vi "GEA2 Message Decoder.vi"(10 "GEA2 Commands and Requests":T9=enum."CMD_WRITE_SETPOINTS", 11 "Coverted Data Out":T10 {"CRC" format="%04x"; "Length" format="%02x"; "Command" format="%02x"; "Destination" format="%02x"; "Source" format="%02x"}) -> (3 "GEA Information Out":T1={"GEA Diagnostic Data - Washer"={"Speed (RPM)"=0, "Load Size"=0, "Temperature"=0, "Water Pressure"=0.0, "Detergent"=0, "Fabric Softener"=0, "Tub Direction"="", "Detergent Valve"=FALSE, "Fabric Softener Valve"=FALSE, "Recirculating Pump"=FALSE, "Drain Valve"=FALSE, "Hot Valve"=FALSE, "Cold Valve"=FALSE, "Lid Closed Status"="", "Lid Lock Status"="", "Error Count"=0, "IGBT Temperature (Deg C)"=0, "Motor Speed"=0, "Latched OOB"=0, "Raw OOB"=0, "Plaster Status"=0, "Inverter Power (W)"=0, "Target Speed(BRPM)"=0, "Latched Agitate Motor Temp (Deg C)"=0, "Current Motor Temp (Deg C)"=0, "Profiler Status"="", "Current Inverter Action"="", "Error Codes"="", "Lid Locked"=FALSE, "Lid Closed"=FALSE, "9E Diagnostic Data"={"Total Cycle Time (Min)"=0, "Total Cycle Count (Current)"=0, "Total Error Count"=0, "Machine Error History"=0, "Washer UI History"=0, "Inverter Error History"=0, "Cycle Storage Limit"=0, "Error Storage Limit"=0, "Cycle Pages Supported"=0, "Error Pages Supported"=0, "Inverter Reset Count"=0}, "9F Diagnostic Data"={"Cycle Buffer Index"="", "Page Number"="", "Total Cycle Count"=0, "Delay Start Time"=0, "Stain Selected"="", "Selected Cycle"=0, "eWash"="", "Soil Level"="", "Temperature"="", "Overnight Ready"="", "Spin Setting"="", "Control Lock Status"="", "Stain Remover"="", "Steam Assist"="", "My Cycle"="", "PreWash"="", "Debug Log Enabled"="", "Rinse"="", "Signal Level"="", "PreSoak"=""}}, "Software Version"={"Critical Major SW Version"="", "Critical Minor SW Version"="", "Major SW Version"="", "Minor SW Version"="", "Parametric Data Ver. Major"="", "Parametric Data Ver. Minor"="", "Diagnostics Data Ver. Major"="", "Diagnostics Data Ver. Minor"="", "Current Personality Setting"=""}, "Debug Search Parameters"={"Pause"=["MchStdby", "MchPz", "MchIdl", "Machine Standby", "Machine Pause", "Machine Idle"], "Run"=["MchRn", "Machine Run", "Resume Process"], "EOC"=["EOC"], "Error Codes"=["Error1", "try", "rty", "inverr"]}, "Message Count"=0, "Number of Messages"=0, "Partial Message String"="", "Full Message to Save"="", "Board ID"="", "Board Index"=0, "Source Address"=0, "Destination Address"=0, "Data to send"=[], "ReceivedData"=[], "Debug/GEA Data"=[], "Command"=0, "GEA2 Reference Out"=refnum, "GEA2 Event Registration"=refnum, "Bus Data"="", "GEA Data"=[], "Network Variable Location"=0, "Water Heater GEA2 Data"={"GEA2 Label Array"=[], "PID_PARAMETERS"=[], "SUPPORTED_MODES"=[], "Button Status"={"Switch 1"=FALSE, "Switch 2"=FALSE, "Switch 3"=FALSE, "Switch 4"=FALSE, "Switch 5"=FALSE, "Switch 6"=FALSE, "Switch 7"=FALSE, "Switch 8"=FALSE, "Switch 9"=FALSE, "Switch 10"=FALSE, "Switch 11"=FALSE, "Switch 12"=FALSE, "Switch 13"=FALSE, "Switch 14"=FALSE, "Switch 15"=FALSE, "Switch 16"=FALSE}, "Status Query"={"Days Remaining (For Std Electric and Vacation)"=0, "Unit Status"="", "Current Tank Temp in Deg F"=0, "Current Setpoint in Deg F"=0, "Filter Status (% used)"=0, "Fallback Status (Fallback heating mode)"="", "Fallback Temp"=0, "\"Set Mode\" Selection"=""}, "Service Error Codes"={"Reserved"=FALSE, "Reserved 1"=FALSE, "Reserved 2"=FALSE, "Reserved 3"=FALSE, "Reserved 4"=FALSE, "Reserved 5"=FALSE, "Reserved 6"=FALSE, "Reserved 7"=FALSE, "DataFlash Fail Status"=FALSE, "Stuck Key Fail Status"=FALSE, "Dry Tank Fail Status"=FALSE, "Miswire Fail Status"=FALSE, "Reserved 8"=FALSE, "Reserved 9"=FALSE, "Reserved 10"=FALSE, "Reserved 11"=FALSE, "UE Fail Status"=FALSE, "LE Fail Status"=FALSE, "Filter Fail Status"=FALSE, "T3A Fail Status"=FALSE, "T3B Fail Status"=FALSE, "T4 Fail Status"=FALSE, "T5 Fail Status"=FALSE, "T2 Fail Status"=FALSE, "SS Cond A Status"=FALSE, "SS Cond B Status"=FALSE, "SS Cond C Status"=FALSE, "SS Cond D Status"=FALSE, "SS Cond E Status"=FALSE, "SS Cond F Status"=FALSE, "SS Fan Status"=FALSE, "CMP Fail Status"=FALSE}, "HEM_KWH_DATA"=[], "OTHER_FAULT_COUNTS"=[], "GEA2 Raw Message"="", "Hyperterminal Data"={"Source"=0, "Destination"=0, "Command"=0, "Length"=0, "CRC"=0, "UE - state (1/0 on off)"=0, "LE - state (1/0 on off)"=0, "Comp - state (1/0 on off)"=0, "Fan  - state (1/0 on off)"=0, "Setpoint Deg F"=0, "T2(TankSensor)"=0.0, "T3A(EvapIn)"=0.0, "T3B(EvapOut)"=0.0, "T4(CompressorDischarge)"=0.0, "T5(Ambient)"=0.0, "Current"=0.0, "Voltage (Volts)"=0, "EEV Position (0-480)"=0, "Reason for last heating cycle termination"=0, "Reason Data word 1"="", "Reason Data word 2"="", "Reason Data word 3"="", "Reason Data word 4"="", "SW Debug Data"="", "Flow Events (Bit Encoded)"=0, "Heating Control Mode"=0}, "Extra Data"={"Water Capacity (Gallons)"=0, "Max Vacation Duration Days"=0, "Min Vacation Duration Days"=0, "Max Set Point (Deg F)"=0, "Min Set Point (Deg F)"=0, "T5 Resistance"=0, "T4 Resistance"=0, "T3B Resistance"=0, "T2 Resistance"=0, "STD_ELEC_RANGE"="", "SS_FAULT_COUNTS"="", "SERIAL_NUMBER"="", "READ_PERSONALITY"=0, "RQST_OVERRIDE_STATUS"="", "MODEL_SELECT_AD_VALUE"=0, "MODEL NUMBER"="", "IDLB_RESISTANCE"=0, "DSM Override Status"="", "RQST_DATA_FROM_Memory"="", "RQST_DATA_FROM_DATA_FLASH"="", "RQST_CURRENT_PID_SH_TARGET"=0, "Unit System Mode"=""}}} {"Water Heater GEA2 Data"."Hyperterminal Data"."CRC" format="%x"; "Water Heater GEA2 Data"."Hyperterminal Data"."Length" format="%x"; "Water Heater GEA2 Data"."Hyperterminal Data"."Command" format="%x"; "Water Heater GEA2 Data"."Hyperterminal Data"."Destination" format="%x"; "Water Heater GEA2 Data"."Hyperterminal Data"."Source" format="%x"; "Destination Address" format="%x"; "Source Address" format="%x"; "Command" format="%.0x"; "Data to send" format="%x"; "ReceivedData" format="%x"})   [LabVIEW 2016]
uses:
  LabVIEW GEA2 Toolkit v1.0.0.0/type defs/Data Out.ctl
  Type Definitions/GEA2 Commands.ctl
  Washer HCC/Washer HCC NEWFI/Type Definitions/ViperHawk/ViperHawk Data.ctl
  Washer HCC/Washer HCC NEWFI/Type Definitions/ViperHawk/ViperHawk Diagnostic Data.ctl
  Save File/Public/Type Definitions/Save File Software Version.ctl
  Washer HCC/Washer HCC NEWFI/Type Definitions/ViperHawk/ViperHawk Search Control.ctl
  C:/TechnologyLab/NI-2010/Trunk/Utility/LabVIEW GEA2 Toolkit v1.0.0.0/Appliance.NET/GeaCommunication.dll
  LabVIEW GEA2 Toolkit v1.0.0.0/Appliance.NET/GeaCommunication.dll
  Type Definitions/GEA2 Commands WaterHeater GEA2 Data.ctl
  Type Definitions/GEA2 Commands Button Status.ctl
  Type Definitions/GEA2 Commands Status Query.ctl
  Type Definitions/GEA2 Commands Service Error Codes.ctl
  LabVIEW GEA2 Toolkit v1.0.0.0/library/GEA2_Toolkit.lvlib
  Save File/Save File.lvlib
panel:
  in  "GEA Information In":T1={"GEA Diagnostic Data - Washer"={"Speed (RPM)"=0, "Load Size"=0, "Temperature"=0, "Water Pressure"=0.0, "Detergent"=0, "Fabric Softener"=0, "Tub Direction"="", "Detergent Valve"=FALSE, "Fabric Softener Valve"=FALSE, "Recirculating Pump"=FALSE, "Drain Valve"=FALSE, "Hot Valve"=FALSE, "Cold Valve"=FALSE, "Lid Closed Status"="", "Lid Lock Status"="", "Error Count"=0, "IGBT Temperature (Deg C)"=0, "Motor Speed"=0, "Latched OOB"=0, "Raw OOB"=0, "Plaster Status"=0, "Inverter Power (W)"=0, "Target Speed(BRPM)"=0, "Latched Agitate Motor Temp (Deg C)"=0, "Current Motor Temp (Deg C)"=0, "Profiler Status"="", "Current Inverter Action"="", "Error Codes"="", "Lid Locked"=FALSE, "Lid Closed"=FALSE, "9E Diagnostic Data"={"Total Cycle Time (Min)"=0, "Total Cycle Count (Current)"=0, "Total Error Count"=0, "Machine Error History"=0, "Washer UI History"=0, "Inverter Error History"=0, "Cycle Storage Limit"=0, "Error Storage Limit"=0, "Cycle Pages Supported"=0, "Error Pages Supported"=0, "Inverter Reset Count"=0}, "9F Diagnostic Data"={"Cycle Buffer Index"="", "Page Number"="", "Total Cycle Count"=0, "Delay Start Time"=0, "Stain Selected"="", "Selected Cycle"=0, "eWash"="", "Soil Level"="", "Temperature"="", "Overnight Ready"="", "Spin Setting"="", "Control Lock Status"="", "Stain Remover"="", "Steam Assist"="", "My Cycle"="", "PreWash"="", "Debug Log Enabled"="", "Rinse"="", "Signal Level"="", "PreSoak"=""}}, "Software Version"={"Critical Major SW Version"="", "Critical Minor SW Version"="", "Major SW Version"="", "Minor SW Version"="", "Parametric Data Ver. Major"="", "Parametric Data Ver. Minor"="", "Diagnostics Data Ver. Major"="", "Diagnostics Data Ver. Minor"="", "Current Personality Setting"=""}, "Debug Search Parameters"={"Pause"=["MchStdby", "MchPz", "MchIdl", "Machine Standby", "Machine Pause", "Machine Idle"], "Run"=["MchRn", "Machine Run", "Resume Process"], "EOC"=["EOC"], "Error Codes"=["Error1", "try", "rty", "inverr"]}, "Message Count"=0, "Number of Messages"=0, "Partial Message String"="", "Full Message to Save"="", "Board ID"="", "Board Index"=0, "Source Address"=0, "Destination Address"=0, "Data to send"=[], "ReceivedData"=[], "Debug/GEA Data"=[], "Command"=0, "GEA2 Reference Out"=refnum, "GEA2 Event Registration"=refnum, "Bus Data"="", "GEA Data"=[], "Network Variable Location"=0, "Water Heater GEA2 Data"={"GEA2 Label Array"=[], "PID_PARAMETERS"=[], "SUPPORTED_MODES"=[], "Button Status"={"Switch 1"=FALSE, "Switch 2"=FALSE, "Switch 3"=FALSE, "Switch 4"=FALSE, "Switch 5"=FALSE, "Switch 6"=FALSE, "Switch 7"=FALSE, "Switch 8"=FALSE, "Switch 9"=FALSE, "Switch 10"=FALSE, "Switch 11"=FALSE, "Switch 12"=FALSE, "Switch 13"=FALSE, "Switch 14"=FALSE, "Switch 15"=FALSE, "Switch 16"=FALSE}, "Status Query"={"Days Remaining (For Std Electric and Vacation)"=0, "Unit Status"="", "Current Tank Temp in Deg F"=0, "Current Setpoint in Deg F"=0, "Filter Status (% used)"=0, "Fallback Status (Fallback heating mode)"="", "Fallback Temp"=0, "\"Set Mode\" Selection"=""}, "Service Error Codes"={"Reserved"=FALSE, "Reserved 1"=FALSE, "Reserved 2"=FALSE, "Reserved 3"=FALSE, "Reserved 4"=FALSE, "Reserved 5"=FALSE, "Reserved 6"=FALSE, "Reserved 7"=FALSE, "DataFlash Fail Status"=FALSE, "Stuck Key Fail Status"=FALSE, "Dry Tank Fail Status"=FALSE, "Miswire Fail Status"=FALSE, "Reserved 8"=FALSE, "Reserved 9"=FALSE, "Reserved 10"=FALSE, "Reserved 11"=FALSE, "UE Fail Status"=FALSE, "LE Fail Status"=FALSE, "Filter Fail Status"=FALSE, "T3A Fail Status"=FALSE, "T3B Fail Status"=FALSE, "T4 Fail Status"=FALSE, "T5 Fail Status"=FALSE, "T2 Fail Status"=FALSE, "SS Cond A Status"=FALSE, "SS Cond B Status"=FALSE, "SS Cond C Status"=FALSE, "SS Cond D Status"=FALSE, "SS Cond E Status"=FALSE, "SS Cond F Status"=FALSE, "SS Fan Status"=FALSE, "CMP Fail Status"=FALSE}, "HEM_KWH_DATA"=[], "OTHER_FAULT_COUNTS"=[], "GEA2 Raw Message"="", "Hyperterminal Data"={"Source"=0, "Destination"=0, "Command"=0, "Length"=0, "CRC"=0, "UE - state (1/0 on off)"=0, "LE - state (1/0 on off)"=0, "Comp - state (1/0 on off)"=0, "Fan  - state (1/0 on off)"=0, "Setpoint Deg F"=0, "T2(TankSensor)"=0.0, "T3A(EvapIn)"=0.0, "T3B(EvapOut)"=0.0, "T4(CompressorDischarge)"=0.0, "T5(Ambient)"=0.0, "Current"=0.0, "Voltage (Volts)"=0, "EEV Position (0-480)"=0, "Reason for last heating cycle termination"=0, "Reason Data word 1"="", "Reason Data word 2"="", "Reason Data word 3"="", "Reason Data word 4"="", "SW Debug Data"="", "Flow Events (Bit Encoded)"=0, "Heating Control Mode"=0}, "Extra Data"={"Water Capacity (Gallons)"=0, "Max Vacation Duration Days"=0, "Min Vacation Duration Days"=0, "Max Set Point (Deg F)"=0, "Min Set Point (Deg F)"=0, "T5 Resistance"=0, "T4 Resistance"=0, "T3B Resistance"=0, "T2 Resistance"=0, "STD_ELEC_RANGE"="", "SS_FAULT_COUNTS"="", "SERIAL_NUMBER"="", "READ_PERSONALITY"=0, "RQST_OVERRIDE_STATUS"="", "MODEL_SELECT_AD_VALUE"=0, "MODEL NUMBER"="", "IDLB_RESISTANCE"=0, "DSM Override Status"="", "RQST_DATA_FROM_Memory"="", "RQST_DATA_FROM_DATA_FLASH"="", "RQST_CURRENT_PID_SH_TARGET"=0, "Unit System Mode"=""}}} {"Water Heater GEA2 Data"."Hyperterminal Data"."CRC" format="%x"; "Water Heater GEA2 Data"."Hyperterminal Data"."Length" format="%x"; "Water Heater GEA2 Data"."Hyperterminal Data"."Command" format="%x"; "Water Heater GEA2 Data"."Hyperterminal Data"."Destination" format="%x"; "Water Heater GEA2 Data"."Hyperterminal Data"."Source" format="%x"; "Destination Address" format="%x"; "Source Address" format="%x"; "Command" format="%.0x"; "Data to send" format="%x"; "ReceivedData" format="%x"}
  out "Hex Array Out":string[](array[string])
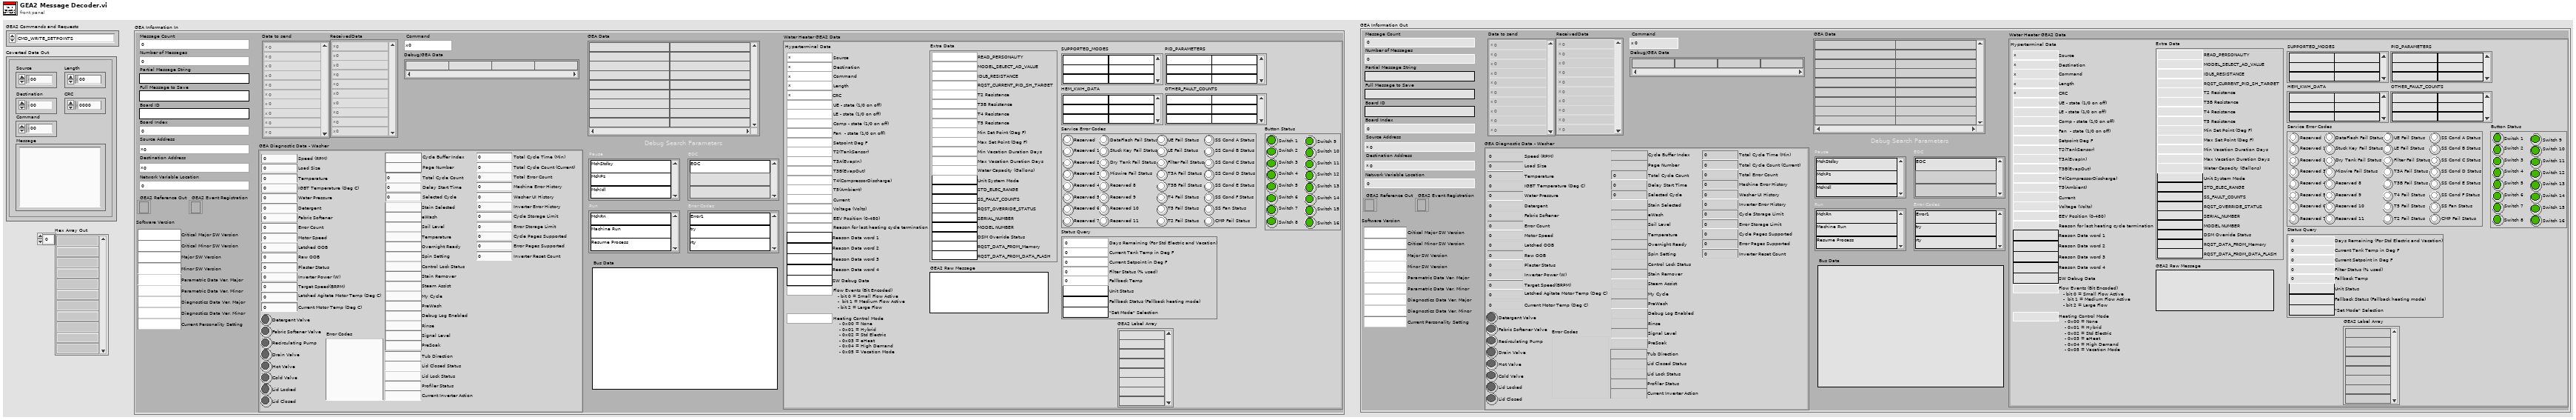
[diagram p1: front panel]
types:
  T1 = typedef "ViperHawk Data.ctl" = cluster{"GEA Diagnostic Data - Washer":T2, "Software Version":T3, "Debug Search Parameters":T4, "Message Count":i32, "Number of Messages":i32, "Partial Message String":string, "Full Message to Save":string, "Board ID":string, "Board Index":i32, "Source Address":u8, "Destination Address":u8, "Data to send":u8[], "ReceivedData":u8[], "Debug/GEA Data":string[], "Command":u8, "GEA2 Reference Out":refnum<k24>, "GEA2 Event Registration":refnum<event-registration>, "Bus Data":string, "GEA Data":string[][], "Network Variable Location":i32, "Water Heater GEA2 Data":T5}
  T2 = typedef "ViperHawk Diagnostic Data.ctl" = cluster{"Speed (RPM)":u32, "Load Size":u32, "Temperature":u32, "Water Pressure":dbl, "Detergent":u32, "Fabric Softener":u32, "Tub Direction":string, "Detergent Valve":bool, "Fabric Softener Valve":bool, "Recirculating Pump":bool, "Drain Valve":bool, "Hot Valve":bool, "Cold Valve":bool, "Lid Closed Status":string, "Lid Lock Status":string, "Error Count":u32, "IGBT Temperature (Deg C)":u32, "Motor Speed":u32, "Latched OOB":u32, "Raw OOB":u32, "Plaster Status":u32, "Inverter Power (W)":u32, "Target Speed(BRPM)":u32, "Latched Agitate Motor Temp (Deg C)":u32, "Current Motor Temp (Deg C)":u32, "Profiler Status":string, "Current Inverter Action":string, "Error Codes":string, "Lid Locked":bool, "Lid Closed":bool, "9E Diagnostic Data":cluster{"Total Cycle Time (Min)":u32, "Total Cycle Count (Current)":u16, "Total Error Count":u16, "Machine Error History":u32, "Washer UI History":u32, "Inverter Error History":u32, "Cycle Storage Limit":u8, "Error Storage Limit":u8, "Cycle Pages Supported":u8, "Error Pages Supported":u8, "Inverter Reset Count":u16}, "9F Diagnostic Data":cluster{"Cycle Buffer Index":string, "Page Number":string, "Total Cycle Count":u32, "Delay Start Time":u32, "Stain Selected":string, "Selected Cycle":u32, "eWash":string, "Soil Level":string, "Temperature":string, "Overnight Ready":string, "Spin Setting":string, "Control Lock Status":string, "Stain Remover":string, "Steam Assist":string, "My Cycle":string, "PreWash":string, "Debug Log Enabled":string, "Rinse":string, "Signal Level":string, "PreSoak":string}}
  T3 = typedef "Save File.lvlib/Save File Software Version.ctl" = cluster{"Critical Major SW Version":string, "Critical Minor SW Version":string, "Major SW Version":string, "Minor SW Version":string, "Parametric Data Ver. Major":string, "Parametric Data Ver. Minor":string, "Diagnostics Data Ver. Major":string, "Diagnostics Data Ver. Minor":string, "Current Personality Setting":string}
  T4 = typedef "ViperHawk Search Control.ctl" = cluster{"Pause":string[], "Run":string[], "EOC":string[], "Error Codes":string[]}
  T5 = typedef "GEA2 Commands WaterHeater GEA2 Data.ctl" = cluster{"GEA2 Label Array":string[], "PID_PARAMETERS":string[][], "SUPPORTED_MODES":string[][], "Button Status":T6, "Status Query":T7, "Service Error Codes":T8, "HEM_KWH_DATA":string[][], "OTHER_FAULT_COUNTS":string[][], "GEA2 Raw Message":string, "Hyperterminal Data":cluster{"Source":u8, "Destination":u8, "Command":u8, "Length":u8, "CRC":u16, "UE - state (1/0 on off)":u8, "LE - state (1/0 on off)":u8, "Comp - state (1/0 on off)":u8, "Fan  - state (1/0 on off)":u8, "Setpoint Deg F":i32, "T2(TankSensor)":dbl, "T3A(EvapIn)":dbl, "T3B(EvapOut)":dbl, "T4(CompressorDischarge)":dbl, "T5(Ambient)":dbl, "Current":dbl, "Voltage (Volts)":u16, "EEV Position (0-480)":u16, "Reason for last heating cycle termination":u16, "Reason Data word 1":string, "Reason Data word 2":string, "Reason Data word 3":string, "Reason Data word 4":string, "SW Debug Data":string, "Flow Events (Bit Encoded)":u16, "Heating Control Mode":u16}, "Extra Data":cluster{"Water Capacity (Gallons)":u32, "Max Vacation Duration Days":u32, "Min Vacation Duration Days":u32, "Max Set Point (Deg F)":u32, "Min Set Point (Deg F)":u32, "T5 Resistance":u32, "T4 Resistance":u32, "T3B Resistance":u32, "T2 Resistance":u32, "STD_ELEC_RANGE":string, "SS_FAULT_COUNTS":string, "SERIAL_NUMBER":string, "READ_PERSONALITY":u8, "RQST_OVERRIDE_STATUS":string, "MODEL_SELECT_AD_VALUE":u32, "MODEL NUMBER":string, "IDLB_RESISTANCE":u32, "DSM Override Status":string, "RQST_DATA_FROM_Memory":string, "RQST_DATA_FROM_DATA_FLASH":string, "RQST_CURRENT_PID_SH_TARGET":u16, "Unit System Mode":string}}
  T6 = typedef "GEA2 Commands Button Status.ctl" = cluster{"Switch 1":bool, "Switch 2":bool, "Switch 3":bool, "Switch 4":bool, "Switch 5":bool, "Switch 6":bool, "Switch 7":bool, "Switch 8":bool, "Switch 9":bool, "Switch 10":bool, "Switch 11":bool, "Switch 12":bool, "Switch 13":bool, "Switch 14":bool, "Switch 15":bool, "Switch 16":bool}
  T7 = typedef "GEA2 Commands Status Query.ctl" = cluster{"Days Remaining (For Std Electric and Vacation)":u8, "Unit Status":string, "Current Tank Temp in Deg F":u8, "Current Setpoint in Deg F":u8, "Filter Status (% used)":u8, "Fallback Status (Fallback heating mode)":string, "Fallback Temp":u8, "\"Set Mode\" Selection":string}
  T8 = typedef "GEA2 Commands Service Error Codes.ctl" = cluster{"Reserved":bool, "Reserved 1":bool, "Reserved 2":bool, "Reserved 3":bool, "Reserved 4":bool, "Reserved 5":bool, "Reserved 6":bool, "Reserved 7":bool, "DataFlash Fail Status":bool, "Stuck Key Fail Status":bool, "Dry Tank Fail Status":bool, "Miswire Fail Status":bool, "Reserved 8":bool, "Reserved 9":bool, "Reserved 10":bool, "Reserved 11":bool, "UE Fail Status":bool, "LE Fail Status":bool, "Filter Fail Status":bool, "T3A Fail Status":bool, "T3B Fail Status":bool, "T4 Fail Status":bool, "T5 Fail Status":bool, "T2 Fail Status":bool, "SS Cond A Status":bool, "SS Cond B Status":bool, "SS Cond C Status":bool, "SS Cond D Status":bool, "SS Cond E Status":bool, "SS Cond F Status":bool, "SS Fan Status":bool, "CMP Fail Status":bool}
  T9 = typedef "GEA2 Commands.ctl" = enum16{"CMD_CANCEL_EEV_POSITION", "CMD_CLEAR_ENERGY_USAGE_CTRS", "CMD_CLEAR_FAULT_COUNTS", "CMD_CLEAR_OVERRIDE_STATUS", "CMD_COMP_OFF", "CMD_COMP_ON", "CMD_DSM_OVERRIDES", "CMD_EEV_POSITION", "CMD_ENTER_EXIT_FCT_MODE", "CMD_ENTER_FACT_MODE", "CMD_HP_RUN_6MIN", "CMD_INITIATE_REMOTE_DSM_OVERRIDE", "CMD_LE_2_SECONDS", "CMD_REFRESH_SERVICE_TIMEOUTS", "CMD_RESET", "CMD_RESET_FILTER_TIMES", "CMD_RESTORE_EEPROM_DEFAULTS", "CMD_RQST_LED_STATUS", "CMD_SET_AMBIENT_THRESH_1", "CMD_SET_AMBIENT_THRESH_2", "CMD_SET_AMBIENT_THRESH_3", "CMD_SET_CURRENTS", "CMD_SET_EEV_DRIVE_LINES", "CMD_SET_EEV_STOP_POSITION", "CMD_SET_LEDS", "CMD_SET_MODEL_NUMBER", "CMD_SET_PID_I_DENOM_OVER_THR", "CMD_SET_PID_I_DENOM_UNDER_THR", "CMD_SET_PID_LOW_SH_TARGET", "CMD_SET_PID_MID_SH_TARGET", "CMD_SET_PID_P_DENOMINATOR", "CMD_SET_SERIAL_NUMBER", "CMD_SET_START_POS_OVER_THR", "CMD_SET_START_POS_UNDER_THR", "CMD_TOGGLE_FAN", "CMD_TOGGLE_LE_SERV", "CMD_TOGGLE_SERVICE_MODE", "CMD_TOGGLE_UE_SERV", "CMD_TURN_ON_OFF_DLB", "CMD_UE_2_SECONDS", "CMD_UPDATE_DSM_LEVEL", "CMD_UPDATE_MODE", "CMD_WRITE_SETPOINTS", "REQ_READ_KEY_STATUS", "REQ_SYSTEM_MODE", "RQST_CURRENT_PID_SH_TARGET", "RQST_DATA_FROM_DATA_FLASH", "RQST_DATA_FROM_MEMORY", "RQST_DSM_OVERRIDE_STATUS", "RQST_HEM_KWH_DATA", "RQST_HYPERTERM_OUTPUT_DATA", "RQST_IDLB_RESISTANCE", "RQST_MODEL_NUMBER", "RQST_MODEL_SELECT_AD_VALUE", "RQST_OTHER_FAULT_COUNTS", "RQST_OVERRIDE_STATUS", "RQST_PID_PARAMETERS", "RQST_READ_PERSONALITY", "RQST_SERIAL_NUMBER", "RQST_SERVICE_ERROR_CODES", "RQST_Software_Version", "RQST_SS_FAULT_COUNTS", "RQST_STATUS_QUERY", "RQST_STD_ELEC_RANGE", "RQST_SUPPORTED_MODES", "RQST_T2_RESISTANCE", "RQST_T3B_RESISTANCE", "RQST_T4_RESISTANCE", "RQST_T5_RESISTANCE", "RQST_TEMP_RANGE", "RQST_VACATION_RANGE", "RQST_WATER_CAPACITY"}
  T10 = typedef "GEA2_Toolkit.lvlib/Data Out.ctl" = cluster{"Source":u8, "Destination":u8, "Command":u8, "Length":u8, "CRC":u16, "Message":string}
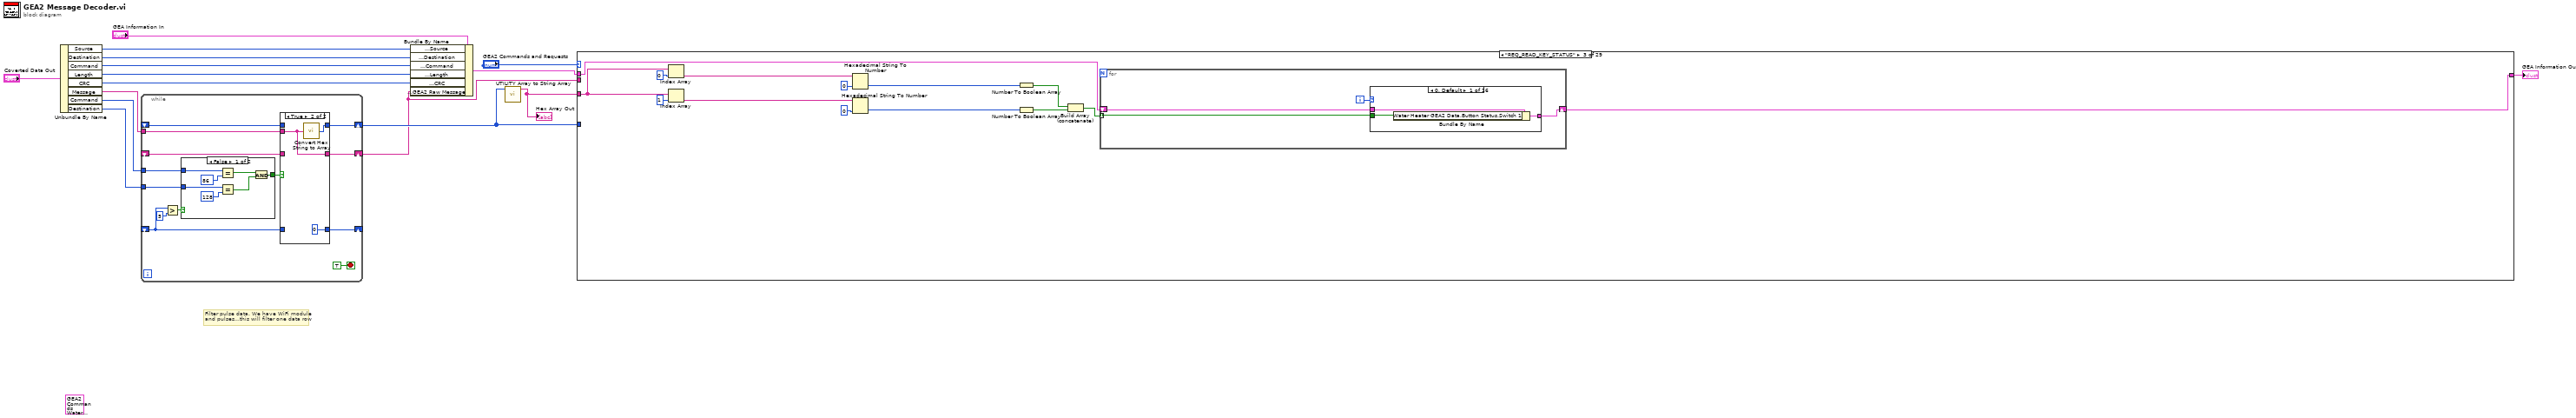
[diagram p0: block diagram]
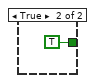
[diagram p2: hidden frame]
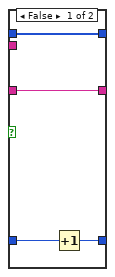
[diagram p3: hidden frame]
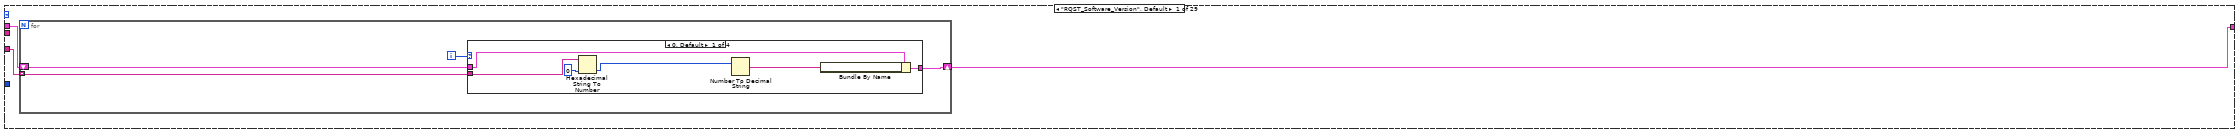
[diagram p4: hidden frame]
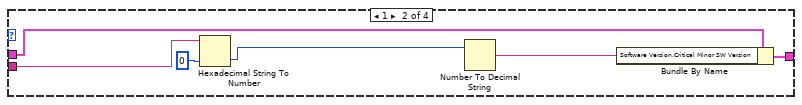
[diagram p5: hidden frame]
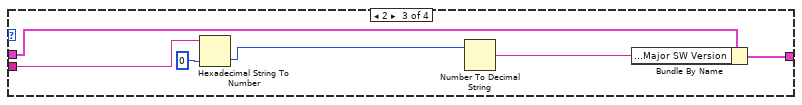
[diagram p6: hidden frame]
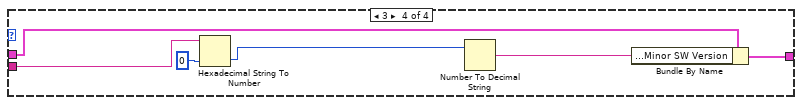
[diagram p7: hidden frame]
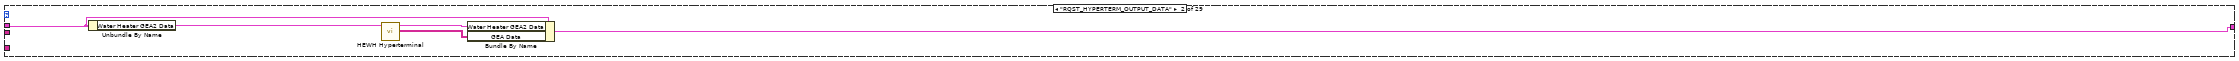
[diagram p8: hidden frame]
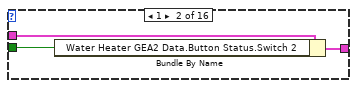
[diagram p9: hidden frame]
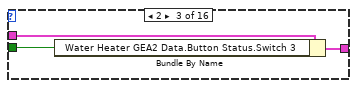
[diagram p10: hidden frame]
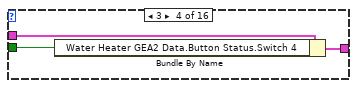
[diagram p11: hidden frame]
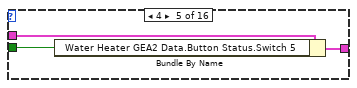
[diagram p12: hidden frame]
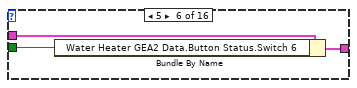
[diagram p13: hidden frame]
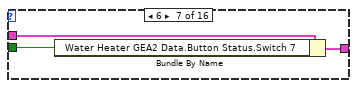
[diagram p14: hidden frame]
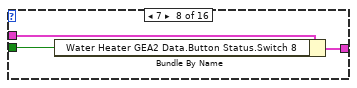
[diagram p15: hidden frame]
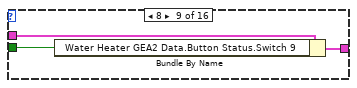
[diagram p16: hidden frame]
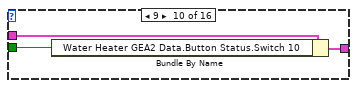
[diagram p17: hidden frame]
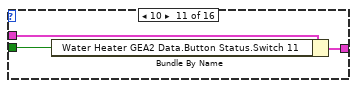
[diagram p18: hidden frame]
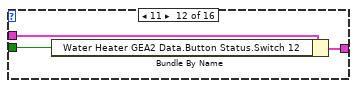
[diagram p19: hidden frame]
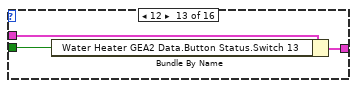
[diagram p20: hidden frame]
diagram:
  (unwired) T5 {"GEA2 Label Array"=[], "PID_PARAMETERS"=[], "SUPPORTED_MODES"=[], "Button Status"={"Switch 1"=FALSE, "Switch 2"=FALSE, "Switch 3"=FALSE, "Switch 4"=FALSE, "Switch 5"=FALSE, "Switch 6"=FALSE, "Switch 7"=FALSE, "Switch 8"=FALSE, "Switch 9"=FALSE, "Switch 10"=FALSE, "Switch 11"=FALSE, "Switch 12"=FALSE, "Switch 13"=FALSE, "Switch 14"=FALSE, "Switch 15"=FALSE, "Switch 16"=FALSE}, "Status Query"={"Days Remaining (For Std Electric and Vacation)"=0, "Unit Status"="", "Current Tank Temp in Deg F"=0, "Current Setpoint in Deg F"=0, "Filter Status (% used)"=0, "Fallback Status (Fallback heating mode)"="", "Fallback Temp"=0, "\"Set Mode\" Selection"=""}, "Service Error Codes"={"Reserved"=FALSE, "Reserved 1"=FALSE, "Reserved 2"=FALSE, "Reserved 3"=FALSE, "Reserved 4"=FALSE, "Reserved 5"=FALSE, "Reserved 6"=FALSE, "Reserved 7"=FALSE, "DataFlash Fail Status"=FALSE, "Stuck Key Fail Status"=FALSE, "Dry Tank Fail Status"=FALSE, "Miswire Fail Status"=FALSE, "Reserved 8"=FALSE, "Reserved 9"=FALSE, "Reserved 10"=FALSE, "Reserved 11"=FALSE, "UE Fail Status"=FALSE, "LE Fail Status"=FALSE, "Filter Fail Status"=FALSE, "T3A Fail Status"=FALSE, "T3B Fail Status"=FALSE, "T4 Fail Status"=FALSE, "T5 Fail Status"=FALSE, "T2 Fail Status"=FALSE, "SS Cond A Status"=FALSE, "SS Cond B Status"=FALSE, "SS Cond C Status"=FALSE, "SS Cond D Status"=FALSE, "SS Cond E Status"=FALSE, "SS Cond F Status"=FALSE, "SS Fan Status"=FALSE, "CMP Fail Status"=FALSE}, "HEM_KWH_DATA"=[], "OTHER_FAULT_COUNTS"=[], "GEA2 Raw Message"="", "Hyperterminal Data"={"Source"=0, "Destination"=0, "Command"=0, "Length"=0, "CRC"=0, "UE - state (1/0 on off)"=0, "LE - state (1/0 on off)"=0, "Comp - state (1/0 on off)"=0, "Fan  - state (1/0 on off)"=0, "Setpoint Deg F"=0, "T2(TankSensor)"=0.0, "T3A(EvapIn)"=0.0, "T3B(EvapOut)"=0.0, "T4(CompressorDischarge)"=0.0, "T5(Ambient)"=0.0, "Current"=0.0, "Voltage (Volts)"=0, "EEV Position (0-480)"=0, "Reason for last heating cycle termination"=0, "Reason Data word 1"="", "Reason Data word 2"="", "Reason Data word 3"="", "Reason Data word 4"="", "SW Debug Data"="", "Flow Events (Bit Encoded)"=0, "Heating Control Mode"=0}, "Extra Data"={"Water Capacity (Gallons)"=0, "Max Vacation Duration Days"=0, "Min Vacation Duration Days"=0, "Max Set Point (Deg F)"=0, "Min Set Point (Deg F)"=0, "T5 Resistance"=0, "T4 Resistance"=0, "T3B Resistance"=0, "T2 Resistance"=0, "STD_ELEC_RANGE"="", "SS_FAULT_COUNTS"="", "SERIAL_NUMBER"="", "READ_PERSONALITY"=0, "RQST_OVERRIDE_STATUS"="", "MODEL_SELECT_AD_VALUE"=0, "MODEL NUMBER"="", "IDLB_RESISTANCE"=0, "DSM Override Status"="", "RQST_DATA_FROM_Memory"="", "RQST_DATA_FROM_DATA_FLASH"="", "RQST_CURRENT_PID_SH_TARGET"=0, "Unit System Mode"=""}}
  # "Filter pulse data. We have WiFi module\nand pulses...this will filter one data row"
  n1 = Unbundle By Name("Coverted Data Out") -> ("Source"=w10:u8, "Destination"=w9:u8, "Command"=w8:u8, "Length"=w7:u8, "CRC"=w6:u16, "Message"=w1:string, "Command"=w4:u8, "Destination"=w3:u8)
  n2 = while {
    shift-right: [w29] -> w5
    shift-left: _ -> [w27]
    tunnel: w4 -> [w22]
    tunnel: w3 -> [w21]
    shift-right: [w25] -> w2
    shift-left: _ -> [w23]
    tunnel: w1 -> [w24]
    shift-right: [w20] -> _
    shift-left: _ -> [w18]
    stop <- TRUE stop-if-true
    n3 = Greater?(x=w18, y=5) -> (0:w19:bool)
    n4 = case shown="False" w19 {
      tunnel: [w34 TRUE] -> w26
      tunnel: w22 -> [w31 _]
      tunnel: w21 -> [w30 _]
      frame False {
        n5 = Equal?(x=w31, y=u8 86) -> (x = y?=w36:bool)
        n6 = Equal?(x=w30, y=u8 128) -> (x = y?=w35:bool)
        n7 = And(x=w36, y=w35) -> (x .and. y?=w34:bool)
      }
      frame True {
      }
    }
    n8 = case shown="True" w26 {
      tunnel: w24 -> [_ w43]
      tunnel: [w41 w44] -> w29
      tunnel: w27 -> [w41 _]
      tunnel: [w40 w43] -> w25
      tunnel: w23 -> [w40 _]
      tunnel: [w39 0] -> w20
      tunnel: w18 -> [w38 _]
      frame False {
        n9 = Increment(x=w38) -> (x+1=w39:i32)
      }
      frame True {
        n10 = call "Convert Hex String to Array.vi"("Hex String In"=w43) -> ("Hex Array Out"=w44:u8[])  [unwired: 14 in]
      }
    }
  }
  n11 = Bundle By Name(cluster="GEA Information In", "Water Heater GEA2 Data.Hyperterminal Data.Source"=w10, "Water Heater GEA2 Data.Hyperterminal Data.Destination"=w9, "Water Heater GEA2 Data.Hyperterminal Data.Command"=w8, "Water Heater GEA2 Data.Hyperterminal Data.Length"=w7, "Water Heater GEA2 Data.Hyperterminal Data.CRC"=w6, "Water Heater GEA2 Data.GEA2 Raw Message"=w2) -> (w11:T1)
  n12 = call "UTILITY Array to String Array.vi"("Hex Array Out"=w5) -> ("Array"=w14:string[])  [unwired: 9 in, 1 out]
  "Hex Array Out" <- w14
  n13 = case shown="\"REQ_READ_KEY_STATUS\"" "GEA2 Commands and Requests" {
    tunnel: w11 -> [w46 w77 w90 w151 w163 w169 w172 w183 w199 w243 w246 w252 w260 w324 w327 w353 w358 w376 w490 w553 w622 w625 w688 w692 w697 w699 w703 w721 w739]
    tunnel: [w45 w79 w81 w147 w157 w167 w170 w176 w198 w242 w244 w250 w259 w322 w325 w351 w356 w362 w488 w552 w620 w623 w686 w690 w694 w698 w702 w719 w736] -> w13
    tunnel: w14 -> [w47 _ w86 _ w162 _ _ w175 w197 w241 _ w253 _ _ w328 _ _ w375 _ w551 _ _ w689 w693 w696 w701 w704 w720 _]
    tunnel: w2 -> [_ _ _ w150 _ w168 w171 _ _ _ _ _ _ w323 _ _ _ _ _ _ w621 _ _ _ _ _ _ _ w738]
    tunnel: w5 -> [_ _ _ _ _ _ _ _ _ _ w249 _ w261 _ _ w355 w359 _ w491 _ _ w628 _ _ _ _ _ _ _]
    frame "RQST_Software_Version", Default {
      n14 = for {
        tunnel: w47 -> [w50] mode=indexing
        shift-right: [w48] -> w45
        shift-left: w46 -> [w49]
        i -> [w51]
        n15 = case shown="0, Default" w51 {
          tunnel: w50 -> [w56 w61 w67 w73]
          tunnel: w49 -> [w55 w63 w68 w74]
          tunnel: [w54 w60 w66 w72] -> w48
          frame 0, Default {
            n16 = Hexadecimal String To Number(string=w56, default (0uL)=u16 0) -> (number=w53:u16)  [unwired: 1 in, 1 out]
            n17 = Number To Decimal String(number=w53) -> (decimal integer string=w52:string)  [unwired: 1 in]
            n18 = Bundle By Name(cluster=w55, "Software Version.Critical Major SW Version"=w52) -> (w54:T1)
          }
          frame 1 {
            n19 = Hexadecimal String To Number(string=w61, default (0uL)=u16 0) -> (number=w59:u16)  [unwired: 1 in, 1 out]
            n20 = Number To Decimal String(number=w59) -> (decimal integer string=w58:string)  [unwired: 1 in]
            n21 = Bundle By Name(cluster=w63, "Software Version.Critical Minor SW Version"=w58) -> (w60:T1)
          }
          frame 2 {
            n22 = Hexadecimal String To Number(string=w67, default (0uL)=u16 0) -> (number=w65:u16)  [unwired: 1 in, 1 out]
            n23 = Number To Decimal String(number=w65) -> (decimal integer string=w64:string)  [unwired: 1 in]
            n24 = Bundle By Name(cluster=w68, "Software Version.Major SW Version"=w64) -> (w66:T1)
          }
          frame 3 {
            n25 = Hexadecimal String To Number(string=w73, default (0uL)=u16 0) -> (number=w71:u16)  [unwired: 1 in, 1 out]
            n26 = Number To Decimal String(number=w71) -> (decimal integer string=w70:string)  [unwired: 1 in]
            n27 = Bundle By Name(cluster=w74, "Software Version.Minor SW Version"=w70) -> (w72:T1)
          }
        }
      }
    }
    frame "RQST_HYPERTERM_OUTPUT_DATA" {
      n28 = Unbundle By Name(w77) -> ("Water Heater GEA2 Data"=w80:T5)
      n29 = call "HEWH Hyperterminal.vi"("Water Heater GEA2 Data In"=w80) -> ("Hyperterminal Data"=w78:string[][], "Water Heater GEA2 Data Out"=w76:T5)  [unwired: 9 in]
      n30 = Bundle By Name(cluster=w77, "Water Heater GEA2 Data"=w76, "GEA Data"=w78) -> (w79:T1)
    }
    frame "REQ_READ_KEY_STATUS" {
      n31 = Index Array(array=w86, index=0) -> (element=w93:string)
      n32 = Index Array(array=w86, index=1) -> (element=w88:string)
      n33 = Hexadecimal String To Number(string=w93, default (0uL)=u8 0 ("default (0 U32)")) -> (number=w91:u8)  [unwired: 1 in, 1 out]
      n34 = Hexadecimal String To Number(string=w88, default (0uL)=u8 0 ("default (0 U32)")) -> (number=w85:u8)  [unwired: 1 in, 1 out]
      n35 = Number To Boolean Array(number=w91) -> (Boolean array=w84:bool[])
      n36 = Number To Boolean Array(number=w85) -> (Boolean array=w83:bool[])
      n37 = Build Array (concatenate)(w84, w83) -> (w82:bool[])
      n38 = for {
        tunnel: w82 -> [w95] mode=indexing
        shift-right: [w96] -> w81
        shift-left: w90 -> [w97]
        i -> [w98]
        n39 = case shown="0, Default" w98 {
          tunnel: w97 -> [w101 w103 w107 w110 w113 w116 w119 w122 w125 w128 w131 w134 w137 w140 w143 w146]
          tunnel: [w100 w104 w106 w109 w112 w115 w118 w121 w124 w127 w130 w133 w136 w139 w142 w145] -> w96
          tunnel: w95 -> [w99 w102 w105 w108 w111 w114 w117 w120 w123 w126 w129 w132 w135 w138 w141 w144]
          frame 0, Default {
            n40 = Bundle By Name(cluster=w101, "Water Heater GEA2 Data.Button Status.Switch 1"=w99) -> (w100:T1)
          }
          frame 1 {
            n41 = Bundle By Name(cluster=w103, "Water Heater GEA2 Data.Button Status.Switch 2"=w102) -> (w104:T1)
          }
          frame 2 {
            n42 = Bundle By Name(cluster=w107, "Water Heater GEA2 Data.Button Status.Switch 3"=w105) -> (w106:T1)
          }
          frame 3 {
            n43 = Bundle By Name(cluster=w110, "Water Heater GEA2 Data.Button Status.Switch 4"=w108) -> (w109:T1)
          }
          frame 4 {
            n44 = Bundle By Name(cluster=w113, "Water Heater GEA2 Data.Button Status.Switch 5"=w111) -> (w112:T1)
          }
          frame 5 {
            n45 = Bundle By Name(cluster=w116, "Water Heater GEA2 Data.Button Status.Switch 6"=w114) -> (w115:T1)
          }
          frame 6 {
            n46 = Bundle By Name(cluster=w119, "Water Heater GEA2 Data.Button Status.Switch 7"=w117) -> (w118:T1)
          }
          frame 7 {
            n47 = Bundle By Name(cluster=w122, "Water Heater GEA2 Data.Button Status.Switch 8"=w120) -> (w121:T1)
          }
          frame 8 {
            n48 = Bundle By Name(cluster=w125, "Water Heater GEA2 Data.Button Status.Switch 9"=w123) -> (w124:T1)
          }
          frame 9 {
            n49 = Bundle By Name(cluster=w128, "Water Heater GEA2 Data.Button Status.Switch 10"=w126) -> (w127:T1)
          }
          frame 10 {
            n50 = Bundle By Name(cluster=w131, "Water Heater GEA2 Data.Button Status.Switch 11"=w129) -> (w130:T1)
          }
          frame 11 {
            n51 = Bundle By Name(cluster=w134, "Water Heater GEA2 Data.Button Status.Switch 12"=w132) -> (w133:T1)
          }
          frame 12 {
            n52 = Bundle By Name(cluster=w137, "Water Heater GEA2 Data.Button Status.Switch 13"=w135) -> (w136:T1)
          }
          frame 13 {
            n53 = Bundle By Name(cluster=w140, "Water Heater GEA2 Data.Button Status.Switch 14"=w138) -> (w139:T1)
          }
          frame 14 {
            n54 = Bundle By Name(cluster=w143, "Water Heater GEA2 Data.Button Status.Switch 15"=w141) -> (w142:T1)
          }
          frame 15 {
            n55 = Bundle By Name(cluster=w146, "Water Heater GEA2 Data.Button Status.Switch 16"=w144) -> (w145:T1)
          }
        }
      }
    }
    frame "REQ_SYSTEM_MODE" {
      n56 = Decimal String To Number(string=w150) -> (number=w149:i32)  [unwired: 2 in, 1 out]
      n57 = case shown="4" w149 {
        tunnel: ["Consumer" "Factory Test" "Service" "Functional Circuit Test" "Demo"] -> w148
        frame 0, Default {
        }
        frame 1 {
        }
        frame 2 {
        }
        frame 3 {
        }
        frame 4 {
        }
      }
      n58 = Bundle By Name(cluster=w151, "Water Heater GEA2 Data.Extra Data.Unit System Mode"=w148) -> (w147:T1)
    }
    frame "RQST_CURRENT_PID_SH_TARGET" {
      n59 = for {
        tunnel: w162 -> [w164] mode=indexing
        shift-right: [w165] -> w160
        shift-left: "" -> [w166]
        n60 = Concatenate Strings(w166, w164) -> (w165:string)
      }
      n61 = Hexadecimal String To Number(string=w160, default (0uL)=u16 0 ("default (0 U32)")) -> (number=w158:u16)  [unwired: 1 in, 1 out]
      n62 = Bundle By Name(cluster=w163, "Water Heater GEA2 Data.Extra Data.RQST_CURRENT_PID_SH_TARGET"=w158) -> (w157:T1)
    }
    frame "RQST_DATA_FROM_DATA_FLASH" {
      n63 = Bundle By Name(cluster=w169, "Water Heater GEA2 Data.Extra Data.RQST_DATA_FROM_DATA_FLASH"=w168) -> (w167:T1)
    }
    frame "RQST_DATA_FROM_MEMORY" {
      n64 = Bundle By Name(cluster=w172, "Water Heater GEA2 Data.Extra Data.RQST_DATA_FROM_Memory"=w171) -> (w170:T1)
    }
    frame "RQST_DSM_OVERRIDE_STATUS" {
      n65 = Delete From Array(array=w175, index=0) -> (array with subset deleted=w173:string[])  [unwired: 1 in, 1 out]
      n66 = for {
        N: 1 -> [_]
        tunnel: w173 -> [w187] mode=indexing
        shift-right: [w188] -> w181
        shift-left: "" -> [w189]
        n67 = Concatenate Strings(w189, w187) -> (w188:string)
      }
      n68 = Hexadecimal String To Number(string=w181, default (0uL)=u16 0 ("default (0 U32)")) -> (number=w178:u16)  [unwired: 1 in, 1 out]
      n69 = case shown="2" w178 {
        tunnel: ["None" "Partial: Override occurred after DSM event started" "Full: Override occurred before DSM event started (auto override)"] -> w177
        frame 0, Default {
        }
        frame 1 {
        }
        frame 2 {
        }
      }
      n70 = Bundle By Name(cluster=w183, "Water Heater GEA2 Data.Extra Data.DSM Override Status"=w177) -> (w176:T1)
    }
    frame "RQST_HEM_KWH_DATA" {
      w205 = 1 ("index")
      n71 = Delete From Array(array=w197, index=0) -> (array with subset deleted=w195:string[])  [unwired: 1 in, 1 out]
      n72 = call "MSB LSB.vi"("Array in"=u8[] [1, 3, 5, 7, 9], "Hex Array Out"=w195) -> ("Array out"=w207:u16[])  [unwired: 9 in]
      n73 = for {
        tunnel: w207 -> [w212]
        tunnel: u8[] [2] -> [w211] mode=indexing
        tunnel: [w210] -> w202
        i -> [w213]
        n74 = case shown="0, Default" w213 {
          tunnel: w212 -> [w216]
          tunnel: w211 -> [w215]
          tunnel: [w217] -> w210
          frame 0, Default {
            n75 = Index Array(array=w216, index=w215) -> (element=w214:u16)
            n76 = Index Array(array=w216, index=1) -> (element=w219:u16)
            n77 = Join Numbers(hi=w219, lo=w214) -> ((hi.lo)=w217:u32)
          }
        }
      }
      n78 = Delete From Array(array=w207, index=w205) -> (array with subset deleted=w206:u16[])  [unwired: 1 in, 1 out]
      n79 = Delete From Array(array=w206, index=w205) -> (array with subset deleted=w204:u16[])  [unwired: 1 in, 1 out]
      n80 = To Unsigned Long Integer(number=w204) -> (unsigned 32bit integer=w203:u32[])
      n81 = Insert Into Array(array=w203, index=1, new element=w202) -> (w200:u32[])
      n82 = for {
        tunnel: w200 -> [w222] mode=indexing
        shift-right: [w220] -> w192
        shift-left: string[] [] -> [w221]
        i -> [w223]
        n83 = case shown="3" w223 {
          tunnel: w222 -> [w227 w231 w235 w239]
          tunnel: [w224 w229 w233 w237] -> w220
          tunnel: w221 -> [w226 w230 w234 w238]
          frame 0, Default {
            n84 = Number To Decimal String(number=w227) -> (decimal integer string=w225:string)  [unwired: 1 in]
            n85 = Build Array (concatenate)(w226, w225) -> (w224:string[])
          }
          frame 1 {
            n86 = Number To Decimal String(number=w231) -> (decimal integer string=w228:string)  [unwired: 1 in]
            n87 = Build Array (concatenate)(w230, w228) -> (w229:string[])
          }
          frame 2 {
            n88 = Number To Decimal String(number=w235) -> (decimal integer string=w232:string)  [unwired: 1 in]
            n89 = Build Array (concatenate)(w234, w232) -> (w233:string[])
          }
          frame 3 {
            n90 = Number To Hexadecimal String(2:w239) -> (0:w236:string)  [unwired: 1 in]
            n91 = Build Array (concatenate)(w238, w236) -> (w237:string[])
          }
        }
      }
      n92 = Build Array(string[] ["Instanteous Power in Watts ", "Watt Seconds used since the last clear ", "Seconds since last clear command ", "Referenced to Line Voltage "], w192) -> (w191:string[][])
      n93 = Transpose 2D Array(2D array=w191) -> (transposed array=w190:string[][])
      n94 = Bundle By Name(cluster=w199, "Water Heater GEA2 Data.HEM_KWH_DATA"=w190) -> (w198:T1)
    }
    frame "RQST_IDLB_RESISTANCE" {
      n95 = call "MSBH_MSBL.vi"("Hex Array Out"=w241) -> ("Value"=w240:u32)  [unwired: 10 in]
      n96 = Bundle By Name(cluster=w243, "Water Heater GEA2 Data.Extra Data.IDLB_RESISTANCE"=w240) -> (w242:T1)
    }
    frame "RQST_MODEL_NUMBER" {
      n97 = Byte Array To String(unsigned byte array=w249) -> (string=w247:string)
      n98 = Match Pattern(string=w247, regular expression="[~0-9]+[0-9]+[A-Z]+") -> (match substring=w245:string)  [unwired: 1 in, 3 out]
      n99 = Bundle By Name(cluster=w246, "Water Heater GEA2 Data.Extra Data.MODEL NUMBER"=w245) -> (w244:T1)
    }
    frame "RQST_MODEL_SELECT_AD_VALUE" {
      n100 = call "MSBH_MSBL.vi"("Hex Array Out"=w253) -> ("Value"=w251:u32)  [unwired: 10 in]
      n101 = Bundle By Name(cluster=w252, "Water Heater GEA2 Data.Extra Data.MODEL_SELECT_AD_VALUE"=w251) -> (w250:T1)
    }
    frame "RQST_OTHER_FAULT_COUNTS" {
      n102 = for {
        tunnel: w261 -> [w262] mode=indexing
        shift-right: [w264] -> w256
        shift-left: string[] [] -> [w265]
        i -> [w263]
        n103 = case shown="0, Default" w263 {
          tunnel: w265 -> [w268 w271 w276 w280 w284 w288 w292 w296 w300 w304 w308 w312 w316 w320]
          tunnel: [w267 w272 w275 w279 w283 w287 w291 w295 w299 w303 w307 w311 w314 w318] -> w264
          tunnel: w262 -> [w269 w273 w277 w281 w285 w289 w293 w297 w301 w305 w309 w313 w317 w321]
          frame 0, Default {
            n104 = Number To Decimal String(number=w269) -> (decimal integer string=w266:string)  [unwired: 1 in]
            n105 = Build Array (concatenate)(w268, w266) -> (w267:string[])
          }
          frame 1 {
            n106 = Number To Decimal String(number=w273) -> (decimal integer string=w270:string)  [unwired: 1 in]
            n107 = Build Array (concatenate)(w271, w270) -> (w272:string[])
          }
          frame 2 {
            n108 = Number To Decimal String(number=w277) -> (decimal integer string=w274:string)  [unwired: 1 in]
            n109 = Build Array (concatenate)(w276, w274) -> (w275:string[])
          }
          frame 3 {
            n110 = Number To Decimal String(number=w281) -> (decimal integer string=w278:string)  [unwired: 1 in]
            n111 = Build Array (concatenate)(w280, w278) -> (w279:string[])
          }
          frame 4 {
            n112 = Number To Decimal String(number=w285) -> (decimal integer string=w282:string)  [unwired: 1 in]
            n113 = Build Array (concatenate)(w284, w282) -> (w283:string[])
          }
          frame 5 {
            n114 = Number To Decimal String(number=w289) -> (decimal integer string=w286:string)  [unwired: 1 in]
            n115 = Build Array (concatenate)(w288, w286) -> (w287:string[])
          }
          frame 6 {
            n116 = Number To Decimal String(number=w293) -> (decimal integer string=w290:string)  [unwired: 1 in]
            n117 = Build Array (concatenate)(w292, w290) -> (w291:string[])
          }
          frame 7 {
            n118 = Number To Decimal String(number=w297) -> (decimal integer string=w294:string)  [unwired: 1 in]
            n119 = Build Array (concatenate)(w296, w294) -> (w295:string[])
          }
          frame 8 {
            n120 = Number To Decimal String(number=w301) -> (decimal integer string=w298:string)  [unwired: 1 in]
            n121 = Build Array (concatenate)(w300, w298) -> (w299:string[])
          }
          frame 9 {
            n122 = Number To Decimal String(number=w305) -> (decimal integer string=w302:string)  [unwired: 1 in]
            n123 = Build Array (concatenate)(w304, w302) -> (w303:string[])
          }
          frame 10 {
            n124 = Number To Decimal String(number=w309) -> (decimal integer string=w306:string)  [unwired: 1 in]
            n125 = Build Array (concatenate)(w308, w306) -> (w307:string[])
          }
          frame 11 {
            n126 = Number To Decimal String(number=w313) -> (decimal integer string=w310:string)  [unwired: 1 in]
            n127 = Build Array (concatenate)(w312, w310) -> (w311:string[])
          }
          frame 12 {
            n128 = Number To Decimal String(number=w317) -> (decimal integer string=w315:string)  [unwired: 1 in]
            n129 = Build Array (concatenate)(w316, w315) -> (w314:string[])
          }
          frame 13 {
            n130 = Number To Decimal String(number=w321) -> (decimal integer string=w319:string)  [unwired: 1 in]
            n131 = Build Array (concatenate)(w320, w319) -> (w318:string[])
          }
        }
      }
      n132 = Build Array(string[] ["Fan Fail Cnt ", "Cmp Fail Cnt ", "UE Fail Cnt ", "LE Fail Cnt ", "Filter Fail Cnt ", "T2 Fail Cnt ", "T3A Fail Cnt ", "T3B Fail Cnt ", "T4 Fail Cnt ", "T5 Fail Cnt ", "DataFlash Fail Cnt ", "Stuck Key Fail Cnt ", "Dry Tank Fail Cnt ", "Miswire Failt Cnt "], w256) -> (w255:string[][])
      n133 = Transpose 2D Array(2D array=w255) -> (transposed array=w254:string[][])
      n134 = Bundle By Name(cluster=w260, "Water Heater GEA2 Data.OTHER_FAULT_COUNTS"=w254) -> (w259:T1)
    }
    frame "RQST_OVERRIDE_STATUS" {
      n135 = Bundle By Name(cluster=w324, "Water Heater GEA2 Data.Extra Data.RQST_OVERRIDE_STATUS"=w323) -> (w322:T1)
    }
    frame "RQST_PID_PARAMETERS" {
      n136 = call "MSB LSB.vi"("Array in"=u8[] [1, 3, 5, 7, 9], "Hex Array Out"=w328) -> ("Array out"=w332:u16[])  [unwired: 9 in]
      n137 = call "MSB LSB.vi"("Array in"=u8[] [11], "Hex Array Out"=w328) -> ("Array out"=w331:u16[])  [unwired: 9 in]
      n138 = for {
        tunnel: u8[] [12, 13, 14, 15, 16] -> [w347] mode=indexing
        tunnel: w328 -> [w348]
        shift-right: [w343] -> w338
        shift-left: string[] [] -> [w344]
        n139 = Index Array(array=w348, index=w347) -> (element=w346:string)
        n140 = Hexadecimal String To Number(string=w346) -> (number=w342:u32)  [unwired: 2 in, 1 out]
        n141 = Number To Decimal String(number=w342) -> (decimal integer string=w345:string)  [unwired: 1 in]
        n142 = Build Array (concatenate)(w344, w345) -> (w343:string[])
      }
      n143 = Build Array (concatenate)(w332, w331) -> (w330:u16[])
      n144 = for {
        tunnel: w330 -> [w350] mode=indexing
        tunnel: [w349] -> w337 mode=indexing
        n145 = Number To Decimal String(number=w350) -> (decimal integer string=w349:string)  [unwired: 1 in]
      }
      n146 = Insert Into Array(array=w337, index=6, new element=w338) -> (w340:string[])
      n147 = Build Array(string[] ["PID P Denominator", "PID I Denominator < Threshold", "PID I Denominator > Threshold", "EEV Start Position < Threshold", "EEV Start Position > Threshold", "EEV Stop Position", "Ambient Temperature Threshold 1", "Ambient Temperature Threshold 2", "Ambient Temperature Threshold 3", "PID Low Running Superheat Target Temperature (deg F)", "PID Mid Running Superheat Target Temperature (deg F)"], w340) -> (w341:string[][])
      n148 = Transpose 2D Array(2D array=w341) -> (transposed array=w326:string[][])
      n149 = Bundle By Name(cluster=w327, "Water Heater GEA2 Data.PID_PARAMETERS"=w326) -> (w325:T1)
    }
    frame "RQST_READ_PERSONALITY" {
      n150 = Index Array(array=w355, index=u8 0) -> (element=w352:u8)
      n151 = Bundle By Name(cluster=w353, "Water Heater GEA2 Data.Extra Data.READ_PERSONALITY"=w352) -> (w351:T1)
    }
    frame "RQST_SERIAL_NUMBER" {
      n152 = Byte Array To String(unsigned byte array=w359) -> (string=w360:string)
      n153 = Match Pattern(string=w360, regular expression="[~0-9]+[0-9]+[A-Z]+") -> (match substring=w357:string)  [unwired: 1 in, 3 out]
      n154 = Bundle By Name(cluster=w358, "Water Heater GEA2 Data.Extra Data.SERIAL_NUMBER"=w357) -> (w356:T1)
    }
    frame "RQST_SERVICE_ERROR_CODES" {
      n155 = Delete From Array(array=w375, index=0) -> (array with subset deleted=w371:string[])  [unwired: 1 in, 1 out]
      n156 = Index Array(array=w371, index=0) -> (element=w386:string)
      n157 = Index Array(array=w371, index=1) -> (element=w382:string)
      n158 = Index Array(array=w371, index=2) -> (element=w366:string)
      n159 = Index Array(array=w371, index=3) -> (element=w365:string)
      n160 = Hexadecimal String To Number(string=w386, default (0uL)=u8 0 ("default (0 U32)")) -> (number=w384:u8)  [unwired: 1 in, 1 out]
      n161 = Hexadecimal String To Number(string=w382, default (0uL)=u8 0 ("default (0 U32)")) -> (number=w380:u8)  [unwired: 1 in, 1 out]
      n162 = Hexadecimal String To Number(string=w366, default (0uL)=u8 0 ("default (0 U32)")) -> (number=w370:u8)  [unwired: 1 in, 1 out]
      n163 = Hexadecimal String To Number(string=w365, default (0uL)=u8 0 ("default (0 U32)")) -> (number=w367:u8)  [unwired: 1 in, 1 out]
      n164 = Number To Boolean Array(number=w384) -> (Boolean array=w379:bool[])
      n165 = Number To Boolean Array(number=w380) -> (Boolean array=w378:bool[])
      n166 = Number To Boolean Array(number=w370) -> (Boolean array=w364:bool[])
      n167 = Number To Boolean Array(number=w367) -> (Boolean array=w363:bool[])
      n168 = Build Array (concatenate)(w379, w378, w364, w363) -> (w377:bool[])
      n169 = for {
        tunnel: w377 -> [w388] mode=indexing
        shift-right: [w389] -> w362
        shift-left: w376 -> [w390]
        i -> [w391]
        n170 = case shown="31" w391 {
          tunnel: w390 -> [w394 w396 w400 w403 w406 w409 w412 w415 w418 w421 w424 w427 w430 w433 w436 w439 w442 w445 w448 w451 w454 w457 w460 w463 w466 w468 w472 w475 w477 w481 w484 w487]
          tunnel: [w393 w397 w399 w402 w405 w408 w411 w414 w417 w420 w423 w426 w429 w432 w435 w438 w441 w444 w447 w450 w453 w456 w459 w462 w465 w467 w471 w474 w478 w480 w483 w486] -> w389
          tunnel: w388 -> [w392 w395 w398 w401 w404 w407 w410 w413 w416 w419 w422 w425 w428 w431 w434 w437 w440 w443 w446 w449 w452 w455 w458 w461 w464 w469 w470 w473 w476 w479 w482 w485]
          frame 0, Default {
            n171 = Bundle By Name(cluster=w394, "Water Heater GEA2 Data.Service Error Codes.Reserved"=w392) -> (w393:T1)
          }
          frame 1 {
            n172 = Bundle By Name(cluster=w396, "Water Heater GEA2 Data.Service Error Codes.Reserved 1"=w395) -> (w397:T1)
          }
          frame 2 {
            n173 = Bundle By Name(cluster=w400, "Water Heater GEA2 Data.Service Error Codes.Reserved 2"=w398) -> (w399:T1)
          }
          frame 3 {
            n174 = Bundle By Name(cluster=w403, "Water Heater GEA2 Data.Service Error Codes.Reserved 3"=w401) -> (w402:T1)
          }
          frame 4 {
            n175 = Bundle By Name(cluster=w406, "Water Heater GEA2 Data.Service Error Codes.Reserved 4"=w404) -> (w405:T1)
          }
          frame 5 {
            n176 = Bundle By Name(cluster=w409, "Water Heater GEA2 Data.Service Error Codes.Reserved 5"=w407) -> (w408:T1)
          }
          frame 6 {
            n177 = Bundle By Name(cluster=w412, "Water Heater GEA2 Data.Service Error Codes.Reserved 6"=w410) -> (w411:T1)
          }
          frame 7 {
            n178 = Bundle By Name(cluster=w415, "Water Heater GEA2 Data.Service Error Codes.Reserved 7"=w413) -> (w414:T1)
          }
          frame 8 {
            n179 = Bundle By Name(cluster=w418, "Water Heater GEA2 Data.Service Error Codes.DataFlash Fail Status"=w416) -> (w417:T1)
          }
          frame 9 {
            n180 = Bundle By Name(cluster=w421, "Water Heater GEA2 Data.Service Error Codes.Stuck Key Fail Status"=w419) -> (w420:T1)
          }
          frame 10 {
            n181 = Bundle By Name(cluster=w424, "Water Heater GEA2 Data.Service Error Codes.Dry Tank Fail Status"=w422) -> (w423:T1)
          }
          frame 11 {
            n182 = Bundle By Name(cluster=w427, "Water Heater GEA2 Data.Service Error Codes.Miswire Fail Status"=w425) -> (w426:T1)
          }
          frame 12 {
            n183 = Bundle By Name(cluster=w430, "Water Heater GEA2 Data.Service Error Codes.Reserved 8"=w428) -> (w429:T1)
          }
          frame 13 {
            n184 = Bundle By Name(cluster=w433, "Water Heater GEA2 Data.Service Error Codes.Reserved 9"=w431) -> (w432:T1)
          }
          frame 14 {
            n185 = Bundle By Name(cluster=w436, "Water Heater GEA2 Data.Service Error Codes.Reserved 10"=w434) -> (w435:T1)
          }
          frame 15 {
            n186 = Bundle By Name(cluster=w439, "Water Heater GEA2 Data.Service Error Codes.Reserved 11"=w437) -> (w438:T1)
          }
          frame 16 {
            n187 = Bundle By Name(cluster=w442, "Water Heater GEA2 Data.Service Error Codes.UE Fail Status"=w440) -> (w441:T1)
          }
          frame 17 {
            n188 = Bundle By Name(cluster=w445, "Water Heater GEA2 Data.Service Error Codes.LE Fail Status"=w443) -> (w444:T1)
          }
          frame 18 {
            n189 = Bundle By Name(cluster=w448, "Water Heater GEA2 Data.Service Error Codes.Filter Fail Status"=w446) -> (w447:T1)
          }
          frame 19 {
            n190 = Bundle By Name(cluster=w451, "Water Heater GEA2 Data.Service Error Codes.T3A Fail Status"=w449) -> (w450:T1)
          }
          frame 20 {
            n191 = Bundle By Name(cluster=w454, "Water Heater GEA2 Data.Service Error Codes.T3B Fail Status"=w452) -> (w453:T1)
          }
          frame 21 {
            n192 = Bundle By Name(cluster=w457, "Water Heater GEA2 Data.Service Error Codes.T4 Fail Status"=w455) -> (w456:T1)
          }
          frame 22 {
            n193 = Bundle By Name(cluster=w460, "Water Heater GEA2 Data.Service Error Codes.T5 Fail Status"=w458) -> (w459:T1)
          }
          frame 23 {
            n194 = Bundle By Name(cluster=w463, "Water Heater GEA2 Data.Service Error Codes.T2 Fail Status"=w461) -> (w462:T1)
          }
          frame 24 {
            n195 = Bundle By Name(cluster=w466, "Water Heater GEA2 Data.Service Error Codes.SS Cond A Status"=w464) -> (w465:T1)
          }
          frame 25 {
            n196 = Bundle By Name(cluster=w468, "Water Heater GEA2 Data.Service Error Codes.SS Cond B Status"=w469) -> (w467:T1)
          }
          frame 26 {
            n197 = Bundle By Name(cluster=w472, "Water Heater GEA2 Data.Service Error Codes.SS Cond C Status"=w470) -> (w471:T1)
          }
          frame 27 {
            n198 = Bundle By Name(cluster=w475, "Water Heater GEA2 Data.Service Error Codes.SS Cond D Status"=w473) -> (w474:T1)
          }
          frame 28 {
            n199 = Bundle By Name(cluster=w477, "Water Heater GEA2 Data.Service Error Codes.SS Cond E Status"=w476) -> (w478:T1)
          }
          frame 29 {
            n200 = Bundle By Name(cluster=w481, "Water Heater GEA2 Data.Service Error Codes.SS Cond F Status"=w479) -> (w480:T1)
          }
          frame 30 {
            n201 = Bundle By Name(cluster=w484, "Water Heater GEA2 Data.Service Error Codes.SS Fan Status"=w482) -> (w483:T1)
          }
          frame 31 {
            n202 = Bundle By Name(cluster=w487, "Water Heater GEA2 Data.Service Error Codes.CMP Fail Status"=w485) -> (w486:T1)
          }
        }
      }
    }
    frame "RQST_SS_FAULT_COUNTS" {
      n203 = for {
        tunnel: w491 -> [w493] mode=indexing
        shift-right: [w495] -> w489
        shift-left: "" -> [w496]
        i -> [w494]
        n204 = case shown="0, Default" w494 {
          tunnel: w496 -> [w497 w505 w510 w516 w524 w529 w534 w540 w546]
          tunnel: [w502 w503 w511 w517 w523 w528 w535 w541 w547] -> w495
          tunnel: w493 -> [w499 w504 w509 w515 w522 w527 w533 w539 w545]
          frame 0, Default {
            n205 = Number To Decimal String(number=w499) -> (decimal integer string=w498:string)  [unwired: 1 in]
            n206 = Concatenate Strings(w497, "SS Cond A Cnt" ("string"), w498, "\r") -> (w502:string)
          }
          frame 1 {
            n207 = Number To Decimal String(number=w504) -> (decimal integer string=w506:string)  [unwired: 1 in]
            n208 = Concatenate Strings(w505, "SS Cond B Cnt" ("string"), w506, "\r") -> (w503:string)
          }
          frame 2 {
            n209 = Number To Decimal String(number=w509) -> (decimal integer string=w512:string)  [unwired: 1 in]
            n210 = Concatenate Strings(w510, "SS Cond C Cnt" ("string"), w512, "\r") -> (w511:string)
          }
          frame 3 {
            n211 = Number To Decimal String(number=w515) -> (decimal integer string=w518:string)  [unwired: 1 in]
            n212 = Concatenate Strings(w516, "SS Cond D Cnt" ("string"), w518, "\r") -> (w517:string)
          }
          frame 4 {
            n213 = Number To Decimal String(number=w522) -> (decimal integer string=w526:string)  [unwired: 1 in]
            n214 = Concatenate Strings(w524, "SS Cond E Cnt" ("string"), w526, "\r") -> (w523:string)
          }
          frame 5 {
            n215 = Number To Decimal String(number=w527) -> (decimal integer string=w532:string)  [unwired: 1 in]
            n216 = Concatenate Strings(w529, "SS Cond F Cnt" ("string"), w532, "\r") -> (w528:string)
          }
          frame 6 {
            n217 = Number To Decimal String(number=w533) -> (decimal integer string=w538:string)  [unwired: 1 in]
            n218 = Concatenate Strings(w534, "SS Cond G Cnt" ("string"), w538, "\r") -> (w535:string)
          }
          frame 7 {
            n219 = Number To Decimal String(number=w539) -> (decimal integer string=w544:string)  [unwired: 1 in]
            n220 = Concatenate Strings(w540, "SS Cond H Cnt" ("string"), w544, "\r") -> (w541:string)
          }
          frame 8 {
            n221 = Number To Decimal String(number=w545) -> (decimal integer string=w550:string)  [unwired: 1 in]
            n222 = Concatenate Strings(w546, "SS Cond I Cnt" ("string"), w550, "\r") -> (w547:string)
          }
        }
      }
      n223 = Bundle By Name(cluster=w490, "Water Heater GEA2 Data.Extra Data.SS_FAULT_COUNTS"=w489) -> (w488:T1)
    }
    frame "RQST_STATUS_QUERY" {
      # "You need to delete the first array\nelement...that is part of the sent message"
      n224 = Delete From Array(array=w551, index=0) -> (array with subset deleted=w554:string[])  [unwired: 1 in, 1 out]
      n225 = for {
        tunnel: w554 -> [w558] mode=indexing
        shift-right: [w556] -> w552
        shift-left: w553 -> [w557]
        i -> [w559]
        n226 = case shown="7" w559 {
          tunnel: w558 -> [w565 w574 w580 w583 w590 w592 w603 w610]
          tunnel: w557 -> [w563 w575 w578 w586 w589 w594 w605 w609]
          tunnel: [w562 w576 w579 w585 w588 w593 w604 w608] -> w556
          frame 0, Default {
            n227 = Hexadecimal String To Number(string=w565, default (0uL)=u8 0 ("default (0 U32)")) -> (number=w564:u8)  [unwired: 1 in, 1 out]
            n228 = case shown="5" w564 {
              tunnel: ["None" "Hybrid" "Std Electric" "eHeat" "High Demand" "Vacation"] -> w561
              frame 0, Default {
              }
              frame 1 {
              }
              frame 2 {
              }
              frame 3 {
              }
              frame 4 {
              }
              frame 5 {
              }
            }
            n229 = Bundle By Name(cluster=w563, "Water Heater GEA2 Data.Status Query.Unit Status"=w561) -> (w562:T1)
          }
          frame 1 {
            n230 = Hexadecimal String To Number(string=w574, default (0uL)=u8 0 ("default (0 U32)")) -> (number=w572:u8)  [unwired: 1 in, 1 out]
            n231 = Bundle By Name(cluster=w575, "Water Heater GEA2 Data.Status Query.Days Remaining (For Std Electric and Vacation)"=w572) -> (w576:T1)
          }
          frame 2 {
            n232 = Hexadecimal String To Number(string=w580, default (0uL)=u8 0 ("default (0 U32)")) -> (number=w577:u8)  [unwired: 1 in, 1 out]
            n233 = Bundle By Name(cluster=w578, "Water Heater GEA2 Data.Status Query.Current Tank Temp in Deg F"=w577) -> (w579:T1)
          }
          frame 3 {
            n234 = Hexadecimal String To Number(string=w583, default (0uL)=u8 0 ("default (0 U32)")) -> (number=w582:u8)  [unwired: 1 in, 1 out]
            n235 = Bundle By Name(cluster=w586, "Water Heater GEA2 Data.Status Query.Current Setpoint in Deg F"=w582) -> (w585:T1)
          }
          frame 4 {
            n236 = Hexadecimal String To Number(string=w590, default (0uL)=u8 0 ("default (0 U32)")) -> (number=w587:u8)  [unwired: 1 in, 1 out]
            n237 = Bundle By Name(cluster=w589, "Water Heater GEA2 Data.Status Query.Filter Status (% used)"=w587) -> (w588:T1)
          }
          frame 5 {
            n238 = Hexadecimal String To Number(string=w592, default (0uL)=u8 0 ("default (0 U32)")) -> (number=w597:u8)  [unwired: 1 in, 1 out]
            n239 = case shown="4" w597 {
              tunnel: ["None" "Hybrid" "Std Electric" "eHeat" "High Demand"] -> w596
              frame 0, Default {
              }
              frame 1 {
              }
              frame 2 {
              }
              frame 3 {
              }
              frame 4 {
              }
            }
            n240 = Bundle By Name(cluster=w594, "Water Heater GEA2 Data.Status Query.Fallback Status (Fallback heating mode)"=w596) -> (w593:T1)
          }
          frame 6 {
            n241 = Hexadecimal String To Number(string=w603, default (0uL)=u8 0 ("default (0 U32)")) -> (number=w606:u8)  [unwired: 1 in, 1 out]
            n242 = Bundle By Name(cluster=w605, "Water Heater GEA2 Data.Status Query.Fallback Temp"=w606) -> (w604:T1)
          }
          frame 7 {
            n243 = Hexadecimal String To Number(string=w610, default (0uL)=u8 0 ("default (0 U32)")) -> (number=w613:u8)  [unwired: 1 in, 1 out]
            n244 = case shown="5" w613 {
              tunnel: ["None" "Hybrid" "Std Electric" "eHeat" "High Demand" "Vacation"] -> w612
              frame 0, Default {
              }
              frame 1 {
              }
              frame 2 {
              }
              frame 3 {
              }
              frame 4 {
              }
              frame 5 {
              }
            }
            n245 = Bundle By Name(cluster=w609, "Water Heater GEA2 Data.Status Query.\"Set Mode\" Selection"=w612) -> (w608:T1)
          }
        }
      }
    }
    frame "RQST_STD_ELEC_RANGE" {
      n246 = Bundle By Name(cluster=w622, "Water Heater GEA2 Data.Extra Data.STD_ELEC_RANGE"=w621) -> (w620:T1)
    }
    frame "RQST_SUPPORTED_MODES" {
      n247 = Index Array(array=w628, index=0) -> (element=w626:u8)
      n248 = Number To Boolean Array(number=w626) -> (Boolean array=w629:bool[])
      n249 = for {
        tunnel: w629 -> [w634] mode=indexing
        shift-right: [w635] -> w631
        shift-left: string[] [] -> [w636]
        i -> [w637]
        n250 = case shown="7" w637 {
          tunnel: w636 -> [w641 w646 w651 w658 w664 w670 w676 w682]
          tunnel: [w640 w644 w652 w657 w662 w669 w675 w681] -> w635
          tunnel: w634 -> [w639 w645 w650 w656 w663 w668 w674 w680]
          frame 0, Default {
            n251 = case shown="True" w639 {
              tunnel: ["Not Supported" "Supported"] -> w638
              frame False {
              }
              frame True {
              }
            }
            n252 = Build Array (concatenate)(w641, w638) -> (w640:string[])
          }
          frame 1 {
            n253 = case shown="True" w645 {
              tunnel: ["Not Supported" "Supported"] -> w647
              frame False {
              }
              frame True {
              }
            }
            n254 = Build Array (concatenate)(w646, w647) -> (w644:string[])
          }
          frame 2 {
            n255 = case shown="True" w650 {
              tunnel: ["Not Supported" "Supported"] -> w653
              frame False {
              }
              frame True {
              }
            }
            n256 = Build Array (concatenate)(w651, w653) -> (w652:string[])
          }
          frame 3 {
            n257 = case shown="True" w656 {
              tunnel: ["Not Supported" "Supported"] -> w659
              frame False {
              }
              frame True {
              }
            }
            n258 = Build Array (concatenate)(w658, w659) -> (w657:string[])
          }
          frame 4 {
            n259 = case shown="True" w663 {
              tunnel: ["Not Supported" "Supported"] -> w665
              frame False {
              }
              frame True {
              }
            }
            n260 = Build Array (concatenate)(w664, w665) -> (w662:string[])
          }
          frame 5 {
            n261 = case shown="True" w668 {
              tunnel: ["Not Supported" "Supported"] -> w671
              frame False {
              }
              frame True {
              }
            }
            n262 = Build Array (concatenate)(w670, w671) -> (w669:string[])
          }
          frame 6 {
            n263 = case shown="True" w674 {
              tunnel: ["Not Supported" "Supported"] -> w677
              frame False {
              }
              frame True {
              }
            }
            n264 = Build Array (concatenate)(w676, w677) -> (w675:string[])
          }
          frame 7 {
            n265 = case shown="True" w680 {
              tunnel: ["Not Supported" "Supported"] -> w683
              frame False {
              }
              frame True {
              }
            }
            n266 = Build Array (concatenate)(w682, w683) -> (w681:string[])
          }
        }
      }
      n267 = Build Array(string[] ["Hybrid", "Std Electric", "eHeat", "High Demand", "Vacation Mode", "Reserved", "Reserved", "Reserved"], w631) -> (w633:string[][])
      n268 = Transpose 2D Array(2D array=w633) -> (transposed array=w624:string[][])
      n269 = Bundle By Name(cluster=w625, "Water Heater GEA2 Data.SUPPORTED_MODES"=w624) -> (w623:T1)
    }
    frame "RQST_T2_RESISTANCE" {
      n270 = call "MSBH_MSBL.vi"("Hex Array Out"=w689) -> ("Value"=w687:u32)  [unwired: 10 in]
      n271 = Bundle By Name(cluster=w688, "Water Heater GEA2 Data.Extra Data.T2 Resistance"=w687) -> (w686:T1)
    }
    frame "RQST_T3B_RESISTANCE" {
      n272 = call "MSBH_MSBL.vi"("Hex Array Out"=w693) -> ("Value"=w691:u32)  [unwired: 10 in]
      n273 = Bundle By Name(cluster=w692, "Water Heater GEA2 Data.Extra Data.T3B Resistance"=w691) -> (w690:T1)
    }
    frame "RQST_T4_RESISTANCE" {
      n274 = call "MSBH_MSBL.vi"("Hex Array Out"=w696) -> ("Value"=w695:u32)  [unwired: 10 in]
      n275 = Bundle By Name(cluster=w697, "Water Heater GEA2 Data.Extra Data.T4 Resistance"=w695) -> (w694:T1)
    }
    frame "RQST_T5_RESISTANCE" {
      n276 = call "MSBH_MSBL.vi"("Hex Array Out"=w701) -> ("Value"=w700:u32)  [unwired: 10 in]
      n277 = Bundle By Name(cluster=w699, "Water Heater GEA2 Data.Extra Data.T5 Resistance"=w700) -> (w698:T1)
    }
    frame "RQST_TEMP_RANGE" {
      n278 = for {
        tunnel: w704 -> [w706] mode=indexing
        shift-right: [w705] -> w702
        shift-left: w703 -> [w707]
        i -> [w708]
        n279 = case shown="1" w708 {
          tunnel: w707 -> [w712 w717]
          tunnel: w706 -> [w711 w714]
          tunnel: [w709 w716] -> w705
          frame 0, Default {
            n280 = Hexadecimal String To Number(string=w711, default (0uL)=u32 0 ("default (0 U32)")) -> (number=w710:u32)  [unwired: 1 in, 1 out]
            n281 = Bundle By Name(cluster=w712, "Water Heater GEA2 Data.Extra Data.Min Set Point (Deg F)"=w710) -> (w709:T1)
          }
          frame 1 {
            n282 = Hexadecimal String To Number(string=w714, default (0uL)=u32 0 ("default (0 U32)")) -> (number=w715:u32)  [unwired: 1 in, 1 out]
            n283 = Bundle By Name(cluster=w717, "Water Heater GEA2 Data.Extra Data.Max Set Point (Deg F)"=w715) -> (w716:T1)
          }
        }
      }
    }
    frame "RQST_VACATION_RANGE" {
      n284 = for {
        tunnel: w720 -> [w723] mode=indexing
        shift-right: [w722] -> w719
        shift-left: w721 -> [w724]
        i -> [w725]
        n285 = case shown="1" w725 {
          tunnel: w724 -> [w729 w734]
          tunnel: w723 -> [w728 w731]
          tunnel: [w726 w733] -> w722
          frame 0, Default {
            n286 = Hexadecimal String To Number(string=w728, default (0uL)=u32 0 ("default (0 U32)")) -> (number=w727:u32)  [unwired: 1 in, 1 out]
            n287 = Bundle By Name(cluster=w729, "Water Heater GEA2 Data.Extra Data.Min Vacation Duration Days"=w727) -> (w726:T1)
          }
          frame 1 {
            n288 = Hexadecimal String To Number(string=w731, default (0uL)=u32 0 ("default (0 U32)")) -> (number=w732:u32)  [unwired: 1 in, 1 out]
            n289 = Bundle By Name(cluster=w734, "Water Heater GEA2 Data.Extra Data.Max Vacation Duration Days"=w732) -> (w733:T1)
          }
        }
      }
    }
    frame "RQST_WATER_CAPACITY" {
      n290 = Hexadecimal String To Number(string=w738) -> (number=w737:u32)  [unwired: 2 in, 1 out]
      n291 = Bundle By Name(cluster=w739, "Water Heater GEA2 Data.Extra Data.Water Capacity (Gallons)"=w737) -> (w736:T1)
    }
  }
  "GEA Information Out" <- w13
